vi "SequenceIndexDeleteUI.vi"(10 "SequenceIndexName":string, 11 "VariableManagerRef in":refnum<vi>) -> (3 "VariableManagerRef out":refnum<vi>)   [LabVIEW 2013]
doc: "Create a confirmation window for deleting a sequence index of the given VariableManager reference."
uses:
  VariableManager/VariableManager.lvclass
  API/VariableManagerAPI.lvlib
panel:
  in  "Cancel":bool
  in  "OK":bool
  out "Display":string
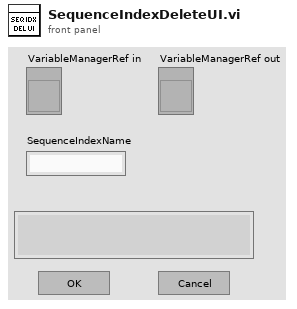
[diagram p1: front panel]
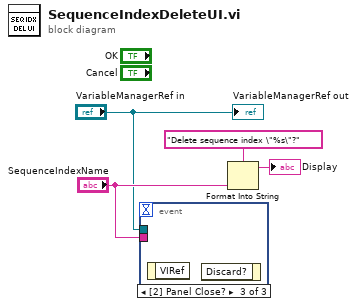
[diagram p0: block diagram]
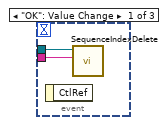
[diagram p2: hidden frame]
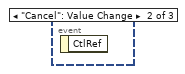
[diagram p3: hidden frame]
diagram:
  n1 = event shown="[2] Panel Close?" {
    selector: _ -> [_ _ _]
    dyn-events: _ -> [_ _ _]
    timeout: _ -> [_ _ _]
    tunnel: "SequenceIndexName" -> [w6 _ _]
    tunnel: "VariableManagerRef in" -> [w5 _ _]
    event "OK": Value Change {
      n2 = event-data() -> ()  [unwired: 1 in, 1 out]
      n3 = call "SequenceIndexDelete.vi"("SequenceIndexName"=w6, "VariableManagerRef in"=w5) -> ()  [unwired: 8 in, 2 out]
    }
    event "Cancel": Value Change {
      n4 = event-data() -> ()  [unwired: 1 in, 1 out]
    }
    event Panel Close? {
      n5 = event-data() -> ()  [unwired: 1 in, 1 out]
      n6 = event-data() -> ()  [unwired: 2 in, 1 out]
    }
  }
  n7 = Format Into String(format string="Delete sequence index \"%s\"?", "SequenceIndexName") -> (resulting string=→"Display":string)  [unwired: 2 in, 1 out]
  "VariableManagerRef out" <- "VariableManagerRef in"
